vi "Set Controller Configuration.vi"(8 "error in (no error)":errorcluster, 11 "Controller in":refnum<class "Controller.lvclass">) -> (0 "error out":errorcluster, 3 "Controller out":refnum<class "Controller.lvclass">)   [LabVIEW 2016, in "Controller Actor.lvlib" / "Controller.lvclass"]
uses:
  Controller.lvclass
  Msmt Configuration/Controller Configuration.lvclass
  <vilib>/Utility/sysdir.llb/System Directory Type.ctl
  Controller.lvclass/Controller.ctl
  Msmt Configuration/Controller Configuration.lvclass/Controller Configuration.ctl
  Msmt Configuration/Read HW Paths.vi
  Msmt Configuration/Read FindHardwareInAppData.vi
  Msmt Configuration/Read Msmt Paths.vi
  Msmt Configuration/Read FindMeasurementsInAppData.vi
  Extensible-Config-Dialog/Configuration.lvclass
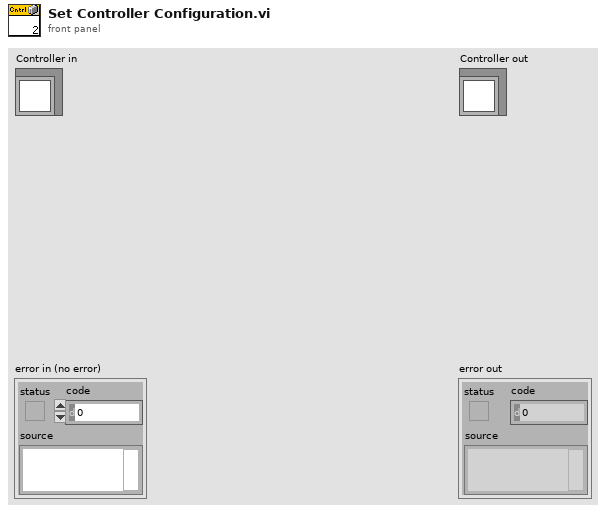
[diagram p1: front panel]
types:
  T1 = typedef "System Directory Type.ctl" = i32
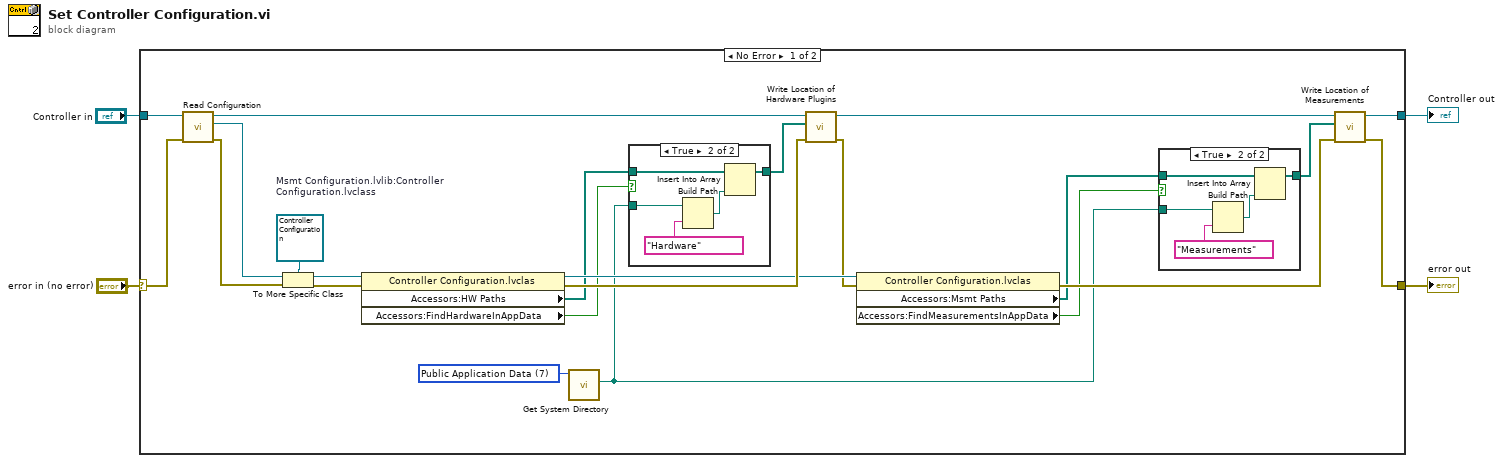
[diagram p0: block diagram]
diagram:
  n1 = case shown="No Error" "error in (no error)" {
    selector: "error in (no error)" -> [w22 w41]
    tunnel: [w23 w41] -> w3
    tunnel: [w25 w40] -> w1
    tunnel: "Controller in" -> [w27 w40]
    frame No Error {
      w12 = T1 7 items=["User Home"=0, "User Desktop"=1, "User Documents"=2, "User Application Data"=3, "User Preferences"=4, "User Temporary"=5, "Public Documents"=6, "Public Application Data"=7, "Public Preferences"=8, "Public Cache"=13, "System Core Libraries"=9, "System Installed Libraries"=10, "Application Files"=11, "Boot Volume Root"=12] ("system directory type")
      w18 = refnum<class "Controller Configuration.lvclass"> refnum  # Msmt Configuration.lvlib:Controller Configuration.lvclass
      n2 = call "Read Configuration.vi"("error in (no error)"=w22, "Controller in"=w27) -> ("error out"=w17:errorcluster, "Configuration.lvlib:Configuration.lvclass"=w16:refnum<class "Configuration.lvclass">, "Controller out"=w26:refnum<class "Controller.lvclass">)  [unwired: 7 in]
      n3 = To More Specific Class(target class=w18, reference=w16, error in=w17) -> (specific class reference=w21:refnum<class "Controller Configuration.lvclass">, error out=w20:errorcluster)
      n4 = property class="Controller Configuration.lvclas"(reference=w21, error in=w20) -> (reference out=w15:refnum<class "Controller Configuration.lvclass">, error out=w19:errorcluster, "Accessors:HW Paths"=w11:path[], "Accessors:FindHardwareInAppData"=w9:bool)
      n5 = call <vilib>:"Get System Directory.vi"("system directory type"=w12) -> ("system directory"=w6:path)  [unwired: 10 in]
      n6 = case shown="True" w9 {
        tunnel: w11 -> [w34 w39]
        tunnel: [w34 w38] -> w10
        tunnel: w6 -> [_ w36]
        frame False {
        }
        frame True {
          n7 = Build Path(base path=w36, name or relative path="Hardware") -> (appended path=w37:path)
          n8 = Insert Into Array(array=w39, new element=w37) -> (w38:path[])  [unwired: 1 in]
        }
      }
      n9 = call "Write Location of Hardware Plugins.vi"("error in (no error)"=w19, "Array of Hardware Paths"=w10, "Controller in"=w26) -> ("error out"=w14:errorcluster, "Controller out"=w24:refnum<class "Controller.lvclass">)  [unwired: 7 in]
      n10 = property class="Controller Configuration.lvclas"(reference=w15, error in=w14) -> (error out=w13:errorcluster, "Accessors:Msmt Paths"=w8:path[], "Accessors:FindMeasurementsInAppData"=w7:bool)  [unwired: 1 out]
      n11 = case shown="True" w7 {
        tunnel: w8 -> [w28 w33]
        tunnel: [w28 w32] -> w5
        tunnel: w6 -> [_ w30]
        frame False {
        }
        frame True {
          n12 = Build Path(base path=w30, name or relative path="Measurements") -> (appended path=w31:path)
          n13 = Insert Into Array(array=w33, new element=w31) -> (w32:path[])  [unwired: 1 in]
        }
      }
      n14 = call "Write Location of Measurements.vi"("error in (no error)"=w13, "Array of Measurements"=w5, "UI Controller in"=w24) -> ("error out"=w23:errorcluster, "UI Controller out"=w25:refnum<class "Controller.lvclass">)  [unwired: 7 in]
    }
    frame Error {
    }
  }
  "error out" <- w3
  "Controller out" <- w1
